vi "VeriPaylasim_Globali.vi"() -> ()   [LabVIEW 2014]
panel:
  in  "FD2 C Fazı Harmonik Ölçüm Değerleri":dbl[](array[numeric])
  in  "FD2 B Fazı Harmonik Ölçüm Değerleri":dbl[](array[numeric])
  in  "FD2 A Fazı Harmonik Ölçüm Değerleri":dbl[](array[numeric])
  in  "FD1 C Fazı Harmonik Ölçüm Değerleri":dbl[](array[numeric])
  in  "FD1 B Fazı Harmonik Ölçüm Değerleri":dbl[](array[numeric])
  in  "FD1 A Fazı Harmonik Ölçüm Değerleri":dbl[](array[numeric])
  in  "Harmonik Limit Değerler":dbl[](array[numeric])
  in  "Uygulanan Değerler":dbl[](array[numeric])
  in  "Uygulanan Değer":dbl
  in  "FD2 C":dbl
  in  "FD2 B":dbl
  in  "FD2 A":dbl
  in  "FD1 C":dbl
  in  "FD1 B":dbl
  in  "FD1 A":dbl
  in  "Limit Deger":dbl
  in  "Ölçüm No":u16
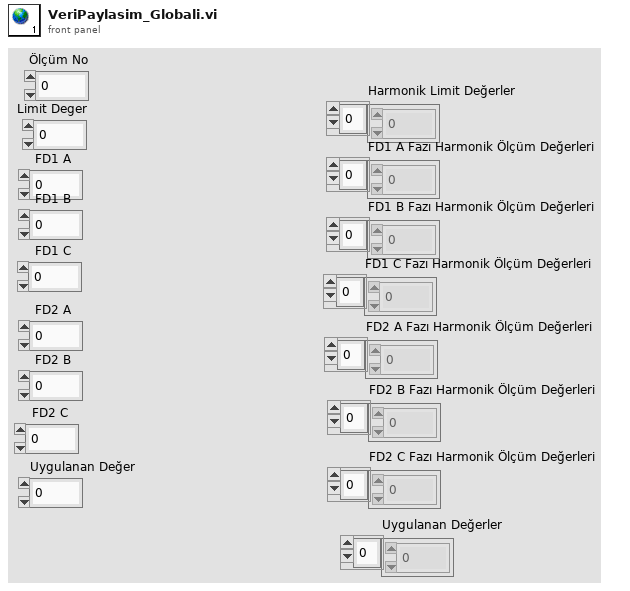
[diagram p1: front panel]
diagram:
